vi "Parent_GetObjectStatus.vi"(0 "reference in":refnum<class "Parent.lvclass">, 5 "error in (no error)":errorcluster) -> (10 "# of objects":i32, 11 "Not a refnum?":bool, 12 "All objects names":string[](array[string]), 13 "Class name":string, 14 "reference out":refnum<class "Parent.lvclass">, 15 "Object name":string, 16 "All refs out":refnum<class "Parent.lvclass">[](array[class]), 19 "error out":errorcluster)   [LabVIEW 2019, in "Parent.lvclass"]
doc: "Returns the object status and also information about all the objects in the class."
uses:
  Parent.lvclass
  protected/ObjectAttributes.ctl
panel:
  in  "DebuggerInput":variant
  out "DebuggerOutput":variant
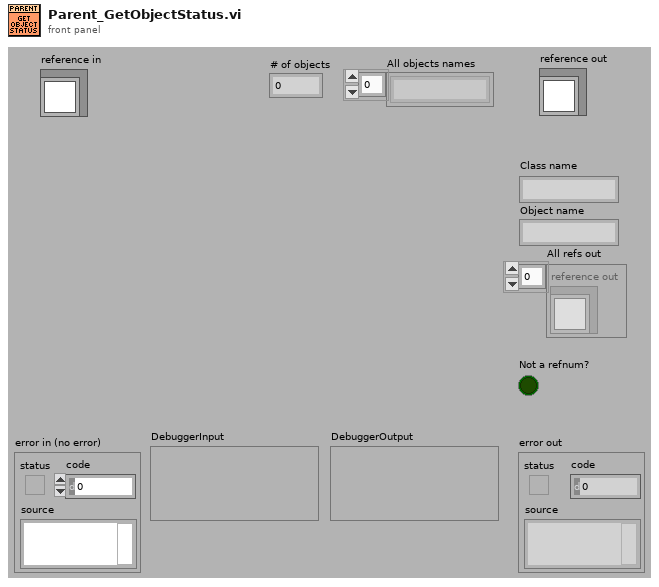
[diagram p1: front panel]
types:
  T1 = typedef "Parent.lvclass/ObjectAttributes.ctl" = cluster{"ParentAttribute":dbl}
  T2 = cluster{"Mode":enum16{"Get", "Set", "Delete"}, "Ref":variant, "ObjAttribute":string, "ClassAttribute":string}
  T3 = cluster{"Object names":string[], "Refs":variant, "ObjectAttributeLocked":bool, "ClassAttributeLocked":bool, "ObjAttribute":variant, "ClassAttribute":variant}
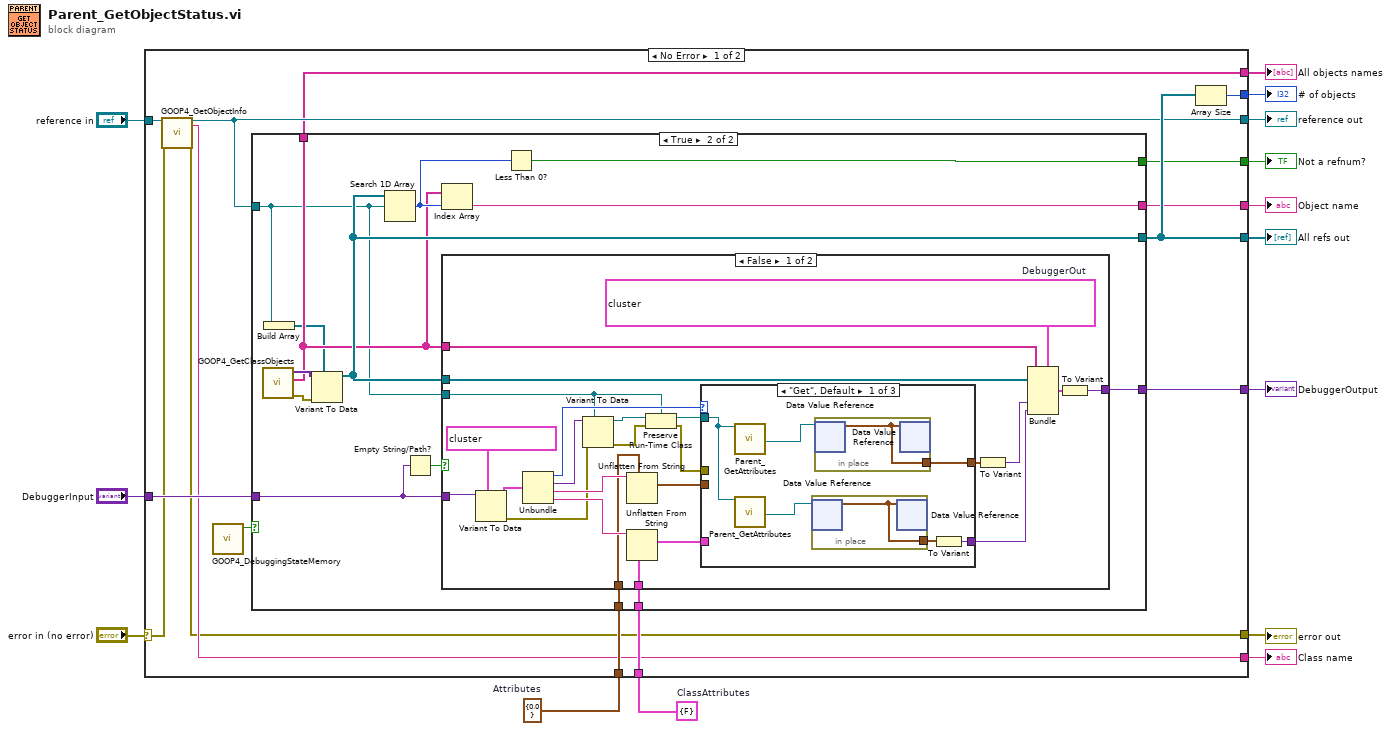
[diagram p0: block diagram]
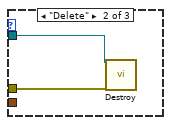
[diagram p3: hidden frame]
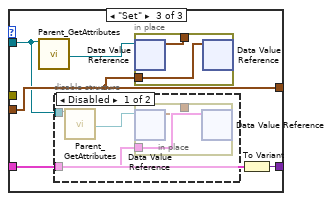
[diagram p4: hidden frame]
diagram:
  w2 = cluster{"classAttribute1":bool} {"classAttribute1"=FALSE}  # ClassAttributes
  w3 = T1 {"ParentAttribute"=0.0}  # Attributes
  n1 = case shown="No Error" "error in (no error)" {
    selector: "error in (no error)" -> [w25 w91]
    tunnel: "reference in" -> [w27 w95]
    tunnel: [w19 w95] -> w12
    tunnel: [w29 -1 ("# of objects")] -> w1
    tunnel: [w17 TRUE ("Exists?")] -> w11
    tunnel: [w22 w92] -> w10
    tunnel: [w15 string[] [] ("Object names")] -> w9
    tunnel: [w18 w92] -> w8
    tunnel: "DebuggerInput" -> [w26 _]
    tunnel: [w28 _] -> w6
    tunnel: [w21 _] -> w5
    tunnel: w3 -> [w24 _]
    tunnel: w2 -> [w23 _]
    tunnel: [w16 w91] -> w4
    frame No Error {
      n2 = call <vilib>:"GOOP4_GetObjectInfo.vi"("ObjectIn"=w27, "error in (no error)"=w25) -> ("ObjectOut"=w19:refnum<class "Parent.lvclass">, "ObjectRuntimeClassName"=w22:string, "error out"=w16:errorcluster)  [unwired: 12 in, 3 out]
      n3 = call <vilib>:"GOOP4_DebuggingStateMemory.vi"() -> ("CurrentDebuggingState"=w20:bool)  [unwired: 10 in, 1 out]
      n4 = case shown="True" w20 {
        tunnel: w26 -> [_ w42]
        tunnel: [_ w41] -> w28
        tunnel: w24 -> [_ w40]
        tunnel: w23 -> [_ w39]
        tunnel: [_ w34] -> w21
        tunnel: [_ w32] -> w15
        tunnel: w19 -> [_ w31]
        tunnel: [_ w36] -> w18
        tunnel: [_ w35] -> w17
        frame False {
        }
        frame True {
          n5 = call <vilib>:"GOOP4_GetClassObjects.vi"() -> ("error out"=w37:errorcluster, "ObjectNames"=w32:string[], "ObjectsRefs"=w38:variant[])  [unwired: 9 in]
          n6 = Build Array(w31) -> (w30:refnum<class "Parent.lvclass">[])
          n7 = Variant To Data(error in=w37, type=w30, Variant=w38) -> (data=w34:refnum<class "Parent.lvclass">[])  [unwired: 1 out]
          n8 = Search 1D Array(1D array=w34, element=w31) -> (index of element=w33:i32)  [unwired: 1 in]
          n9 = Empty String/Path?(string/path=w42) -> (empty?=w43:bool)
          n10 = Index Array(array=w32, index=w33) -> (element=w36:string)
          n11 = case shown="False" w43 {
            tunnel: [w45 _] -> w41
            tunnel: w40 -> [w65 _]
            tunnel: w39 -> [w64 _]
            tunnel: w42 -> [w57 _]
            tunnel: w34 -> [w53 _]
            tunnel: w32 -> [w59 _]
            tunnel: w31 -> [w52 _]
            frame False {
              w58 = T3 {"Object names"=[], "Refs"=variant, "ObjectAttributeLocked"=FALSE, "ClassAttributeLocked"=FALSE, "ObjAttribute"=variant, "ClassAttribute"=variant}  # DebuggerOut
              n12 = Variant To Data(type=T2 {"Mode"=enum."Delete", "Ref"=variant, "ObjAttribute"="", "ClassAttribute"=""} ("DebuggerIn"), Variant=w57) -> (data=w55:T2, error out=w47:errorcluster)  [unwired: 1 in]
              n13 = Unbundle(w55) -> ("Mode"=w63:enum16{"Get", "Set", "Delete"}, "Ref"=w54:variant, "ObjAttribute"=w67:string, "ClassAttribute"=w68:string)
              n14 = Variant To Data(error in=w47, type=w52, Variant=w54) -> (data=w51:refnum<class "Parent.lvclass">, error out=w49:errorcluster)
              n15 = Unflatten From String(type=w65, binary string=w67) -> (value=w66:T1)  [unwired: 3 in, 2 out]
              n16 = Unflatten From String(type=w64, binary string=w68) -> (value=w62:cluster{"classAttribute1":bool})  [unwired: 3 in, 2 out]
              n17 = Preserve Run-Time Class(object in=w51, error in=w49, 2:w52) -> (object out=w50:refnum<class "Parent.lvclass">, error out=w48:errorcluster)
              n18 = case shown="\"Get\", Default" w63 {
                tunnel: w50 -> [w72 w78 w79]
                tunnel: [w74 _ w82] -> w60
                tunnel: [w69 _ w81] -> w44
                tunnel: w66 -> [_ _ w82]
                tunnel: w62 -> [_ _ w80]
                tunnel: w48 -> [_ w77 _]
                frame "Get", Default {
                  n19 = call "Parent_GetAttributes.vi"("reference in"=w72) -> ("DataRef"=w73:refnum<data-value>)  [unwired: 15 in, 3 out]
                  n20 = call "Parent_GetAttributes.vi"("reference in"=w72) -> ("DataRef"=w71:refnum<data-value>)  [unwired: 15 in, 3 out]
                  n21 = in-place {
                    in-place-border: [w75] -> w70
                    n22 = in-place-dvr #1(w71) -> (w75:T1)  [unwired: 1 out]
                    n23 = in-place-dvr #1(w75) -> ()  [unwired: 2 out]
                  }
                  n24 = in-place {
                    in-place-border: [w76] -> w74
                    n25 = in-place-dvr #2(w73) -> (w76:T1)  [unwired: 1 out]
                    n26 = in-place-dvr #2(w76) -> ()  [unwired: 2 out]
                  }
                  n27 = To Variant(anything=w70) -> (Variant=w69:variant)
                }
                frame "Delete" {
                  n28 = call-dynamic "Destroy.vi"("reference in"=w78, "error in (no error)"=w77) -> ()  [unwired: 16 in, 2 out]
                }
                frame "Set" {
                  n29 = call "Parent_GetAttributes.vi"("reference in"=w79) -> ("DataRef"=w83:refnum<data-value>)  [unwired: 15 in, 3 out]
                  n30 = disable-structure shown="Disabled" {
                    disable-tunnel: w80 -> [w85 _]
                    disable-tunnel: w79 -> [w84 _]
                    frame Disabled {
                      n31 = call "Parent_GetAttributes.vi"("reference in"=w84) -> ("DataRef"=w86:refnum<data-value>)  [unwired: 15 in, 3 out]
                      n32 = in-place {
                        in-place-border: w85 -> [w88]
                        in-place-border: [w87] -> _
                        n33 = in-place-dvr #3(w86) -> (w87:T1)  [unwired: 1 out]
                        n34 = in-place-dvr #3(w88) -> ()  [unwired: 2 out]
                      }
                    }
                    frame Enabled {
                    }
                  }
                  n35 = in-place {
                    in-place-border: w82 -> [w90]
                    in-place-border: [w89] -> _
                    n36 = in-place-dvr #4(w83) -> (w89:T1)  [unwired: 1 out]
                    n37 = in-place-dvr #4(w90) -> ()  [unwired: 2 out]
                  }
                  n38 = To Variant(anything=w80) -> (Variant=w81:variant)
                }
              }
              n39 = To Variant(anything=w60) -> (Variant=w61:variant)
              n40 = Bundle(cluster=w58, "Object names"=w59, "Refs"=w53, "ObjAttribute"=w61, "ClassAttribute"=w44) -> (w46:T3)  [unwired: 2 in]
              n41 = To Variant(anything=w46) -> (Variant=w45:variant)
            }
            frame True {
            }
          }
          n42 = Less Than 0?(x=w33) -> (x < 0?=w35:bool)
        }
      }
      n43 = Array Size(array=w21) -> (size(s)=w29:i32)
    }
    frame Error {
      w92 = "" ("Class name")
      (unwired) FALSE
    }
  }
  "error out" <- w4
  "reference out" <- w12
  "# of objects" <- w1
  "Not a refnum?" <- w11
  "All refs out" <- w5
  "Class name" <- w10
  "All objects names" <- w9
  "Object name" <- w8
  "DebuggerOutput" <- w6
